vi "cluster.vi"() -> ()   [LabVIEW 2020]
uses:
  Control 1.ctl
panel:
  out "XY Graph":cluster{dbl[], dbl[]}[](graph)
  out "output cluster":T1
  out "Boolean":bool
  in  "Cluster":T2
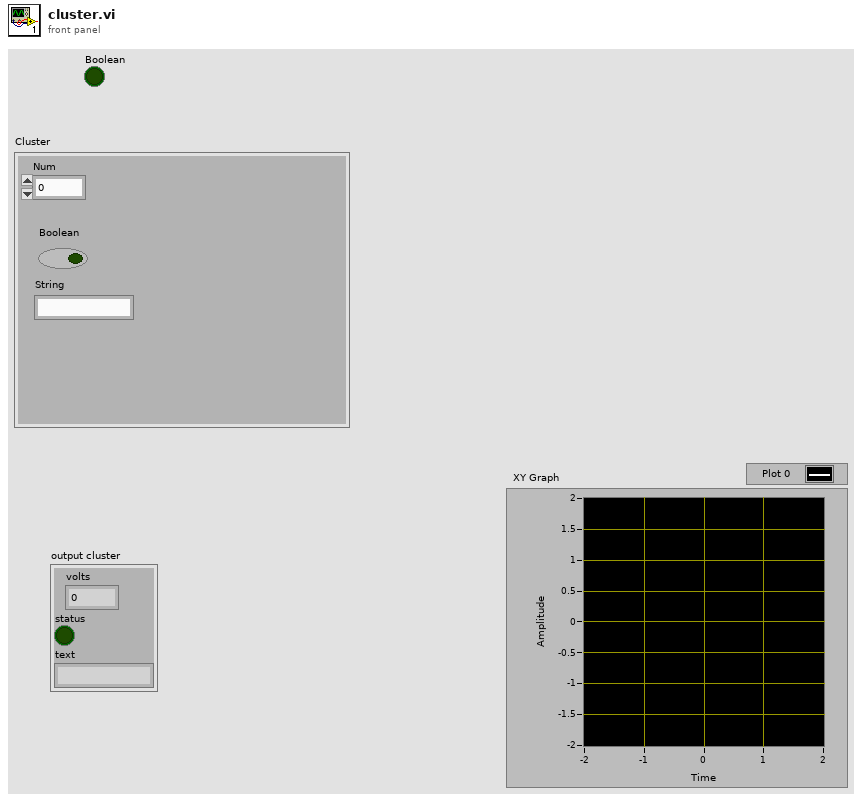
[diagram p1: front panel]
types:
  T1 = cluster{"volts":dbl, "status":bool, "text":string}
  T2 = typedef "Control 1.ctl" = cluster{"String":string, "Num\n":dbl, "Boolean":bool}
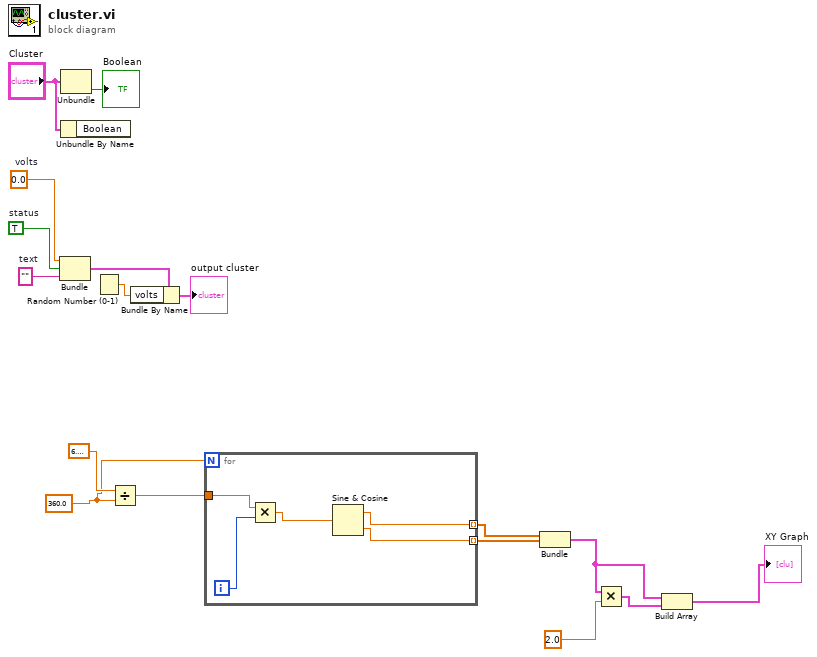
[diagram p0: block diagram]
diagram:
  w8 = 360.0 ("y")
  w14 = ""  # text
  w15 = TRUE  # status
  w16 = 0.0  # volts
  n1 = Bundle("volts"=w16, "status"=w15, "text"=w14) -> (w12:T1)  [unwired: 1 in]
  n2 = Unbundle("Cluster") -> ("Boolean"=→"Boolean":bool)  [unwired: 2 out]
  n3 = Unbundle By Name("Cluster") -> ()  [unwired: 1 out]
  n4 = Random Number (0-1)() -> (number: 0 to 1=w13:dbl)
  n5 = Divide(x=6.283185307179586, y=w8) -> (x/y=w7:dbl)
  n6 = Bundle By Name(cluster=w12, "volts"=w13) -> (→"output cluster":T1)
  n7 = for {
    N: w8 -> [_]
    tunnel: w7 -> [w22]
    tunnel: [w19] -> w6 mode=indexing
    tunnel: [w18] -> w5 mode=indexing
    i -> [w21]
    n8 = Multiply(x=w22, y=w21) -> (x*y=w20:dbl)
    n9 = Sine & Cosine(0:w20) -> (1:w19:dbl, 2:w18:dbl)
  }
  n10 = Bundle(w6, w5) -> (w3:cluster{dbl[], dbl[]})  [unwired: 1 in]
  n11 = Multiply(x=w3, y=2.0) -> (x*y=w4:cluster{dbl[], dbl[]})
  n12 = Build Array(w3, w4) -> (→"XY Graph":cluster{dbl[], dbl[]}[])
